vi "Get SW LRMS.vi"(8 "error in":errorcluster, 11 "cPAS Data in":refnum<class "cPAS Data.lvclass">) -> (0 "error out":errorcluster, 3 "cPAS Data out":refnum<class "cPAS Data.lvclass">)   [LabVIEW 2015, in "cPAS Data.lvclass"]
doc: "Calculate the RMS value of the photodiode signal."
uses:
  cPAS Data.lvclass
  cPAS Cell Data/cPAS Cell Data.lvclass
  <vilib>/Analysis/5stat.llb/RMS (DBL).vi
  Reusable/PAS/Data/Main/Read CellData.vi
  Reusable/PAS/Data/Cell/Read lasDiodeData.vi
  cPAS Cell Data/Write lRMS_hw.vi
  Reusable/PAS/Data/Main/Write CellData.vi
  Reusable/PAS/Data/Cell/PAS Cell Data.lvclass
  <vilib>/Analysis/NI_AALPro.lvlib
panel:
  out "sw_lrms":dbl[](array[numeric])
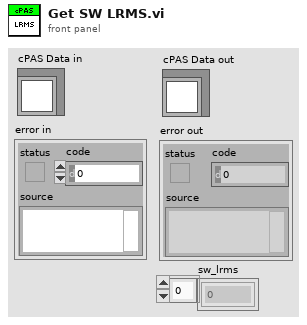
[diagram p1: front panel]
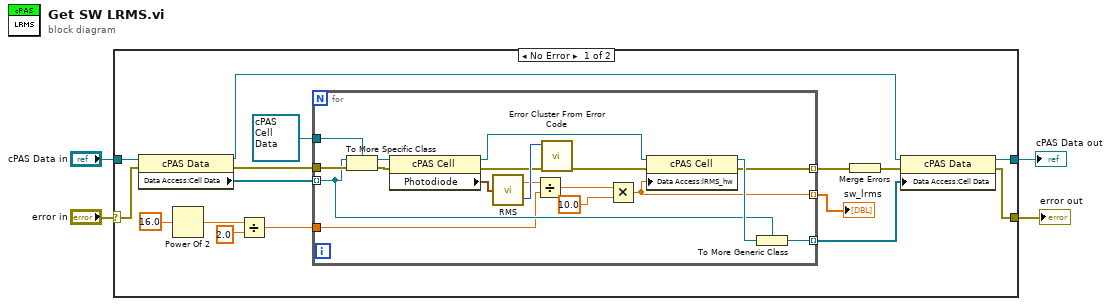
[diagram p0: block diagram]
diagram:
  n1 = case shown="No Error" "error in" {
    selector: "error in" -> [w19 w40]
    tunnel: [w11 w40] -> w3
    tunnel: [w12 w39] -> w1
    tunnel: "cPAS Data in" -> [w20 w39]
    frame No Error {
      n2 = property class="cPAS Data"(reference=w20, error in=w19) -> (reference out=w16:refnum<class "cPAS Data.lvclass">, error out=w6:errorcluster, "Data Access:Cell Data"=w18:refnum<class "PAS Cell Data.lvclass">[])
      n3 = Power Of 2(x=16.0) -> (2^x=w9:dbl)
      n4 = Divide(x=w9, y=2.0) -> (x/y=w5:dbl)
      n5 = for {
        tunnel: w18 -> [w27] mode=indexing
        tunnel: refnum<class "cPAS Cell Data.lvclass"> refnum ("cPAS Cell") -> [w36]
        tunnel: w6 -> [w34]
        tunnel: [w28] -> w15 mode=indexing
        tunnel: [w26] -> w14 mode=indexing
        tunnel: w5 -> [w25]
        tunnel: [w22] -> w7 mode=indexing
        n6 = To More Specific Class(target class=w36, reference=w27, error in=w34) -> (specific class reference=w35:refnum<class "cPAS Cell Data.lvclass">, error out=w33:errorcluster)
        n7 = property class="cPAS Cell"(reference=w35, error in=w33) -> (reference out=w37:refnum<class "cPAS Cell Data.lvclass">, error out=w31:errorcluster, "Photodiode"=w38:waveform(i16))
        n8 = call-poly <vilib>:"RMS.vi"("X"=w38) -> ("rms value"=w21:dbl, "error"=w32:i32)
        n9 = Divide(x=w21, y=w25) -> (x/y=w24:dbl)
        n10 = call <vilib>:"Error Cluster From Error Code.vi"("error in (no error)"=w31, "error code (0)"=w32) -> ("error out"=w30:errorcluster)  [unwired: 7 in]
        n11 = Multiply(x=w24, y=10.0) -> (x*y=w22:dbl)
        n12 = property class="cPAS Cell"(reference=w37, error in=w30, "Data Access:lRMS_hw"=w22) -> (reference out=w29:refnum<class "cPAS Cell Data.lvclass">, error out=w26:errorcluster)
        n13 = To More Generic Class(target class=w27, reference=w29) -> (generic class reference=w28:refnum<class "PAS Cell Data.lvclass">)
      }
      "sw_lrms" <- w7
      n14 = Merge Errors(w14) -> (w13:errorcluster)
      n15 = property class="cPAS Data"(reference=w16, error in=w13, "Data Access:Cell Data"=w15) -> (reference out=w12:refnum<class "cPAS Data.lvclass">, error out=w11:errorcluster)
    }
    frame Error {
    }
  }
  "error out" <- w3
  "cPAS Data out" <- w1
